vi "Angle_init.vi"   [LabVIEW 2019]
uses:
  Global/Global Variables/Data_Display_global.vi
  Global/Global Variables/global.vi
types:
  T1 = typedef "TMCCluster.ctl" = cluster{"Winkel Setpoint":dbl, "Ausgelesener Winkel":dbl, "Aktuelle Position als 0° Setzen":bool, "Da ist was verkehrt!":bool, "Winkel setzen":bool}
  T2 = typedef "TMC_Control.ctl" = cluster{"Winkel Setpoint":dbl, "Aktuelle Position als 0° Setzen":bool, "Winkel setzen":bool}
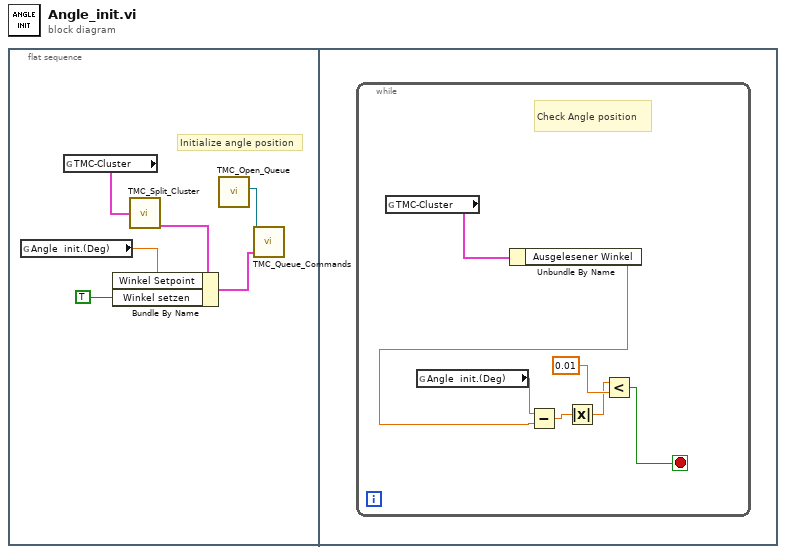
[diagram p0: block diagram]
diagram:
  n1 = flat-sequence {
    frame #0 {
      # "Initialize angle position"
      n2 = global read "global.vi" "Angle  init.(Deg)"() -> (w1:dbl)
      n3 = global read "Data_Display_global.vi" "TMC-Cluster"() -> (w5:T1)
      n4 = call "TMC_Split_Cluster.vi"("TMC Cluster"=w5) -> ("TMC-Control"=w4:T2)  [unwired: 2 in, 1 out]
      n5 = Bundle By Name(cluster=w4, "Winkel Setpoint"=w1, "Winkel setzen"=TRUE) -> (w3:T2)
      n6 = call "TMC_Open_Queue.vi"() -> ("queue out"=w6:refnum<queue>)  [unwired: 10 in, 1 out]
      n7 = call "TMC_Queue_Commands.vi"("TMC-Control"=w3, "TMC Queue"=w6) -> ()  [unwired: 1 in, 1 out]
    }
    frame #1 {
      n8 = while {
        stop <- w11 stop-if-true
        # "Check Angle position"
        n9 = global read "Data_Display_global.vi" "TMC-Cluster"() -> (w8:T1)
        n10 = global read "global.vi" "Angle  init.(Deg)"() -> (w13:dbl)
        n11 = Unbundle By Name(w8) -> ("Ausgelesener Winkel"=w7:dbl)
        n12 = Subtract(x=w13, y=w7) -> (x-y=w10:dbl)
        n13 = Absolute Value(x=w10) -> (abs(x)=w9:dbl)
        n14 = Less?(x=w9, y=0.01) -> (x < y?=w11:bool)
      }
    }
  }
